vi "HEWH Search For Previous Draw Stats.vi"(8 "Error In":errorcluster, 11 "RTD Max Min Array":string[][](array[string])) -> (0 "Error Out":errorcluster, 3 "Previous Draw Stat Index (Row)":i32)   [LabVIEW 2016]
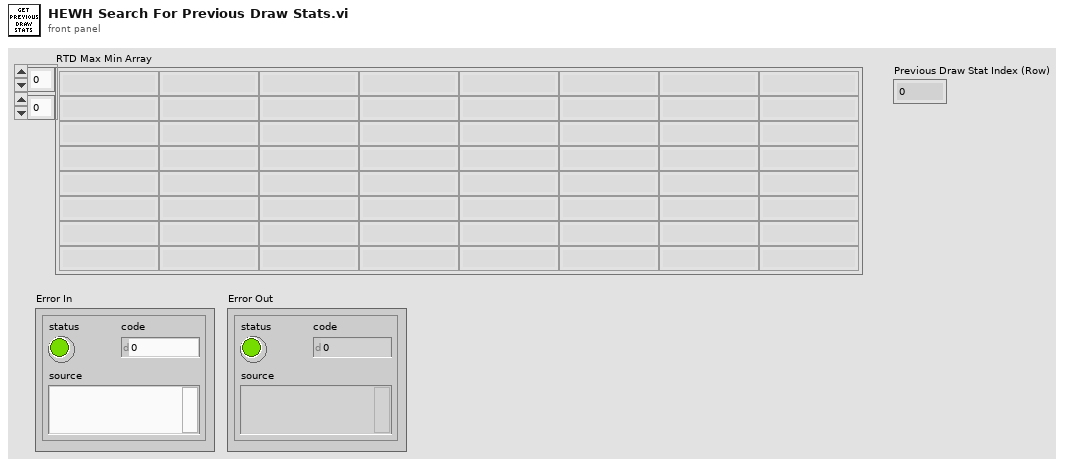
[diagram p1: front panel]
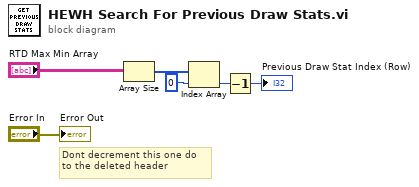
[diagram p0: block diagram]
diagram:
  # "Dont decrement this one do\nto the deleted header"
  n1 = Array Size(array="RTD Max Min Array") -> (size(s)=w4:i32[])
  n2 = Index Array(array=w4, index=0) -> (element=w2:i32)
  n3 = Decrement(x=w2) -> (x-1=→"Previous Draw Stat Index (Row)":i32)
  "Error Out" <- "Error In"
